vi "toggleShutter_v2.vi"(7 "Error In":errorcluster) -> (0 "error out":errorcluster)   [LabVIEW 2021]
doc: "Newport Motion Controler\nThis program Toggle Shutter (open / close)\n\nAndré Romero - 2020\nandretec@ifsc.usp.br"
uses:
  Global Shutter.vi
panel:
  out "VISA Refnum out":refnum<visa-resource-name>
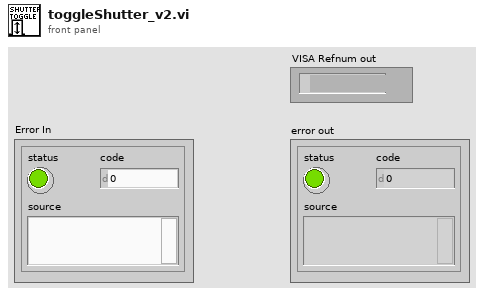
[diagram p1: front panel]
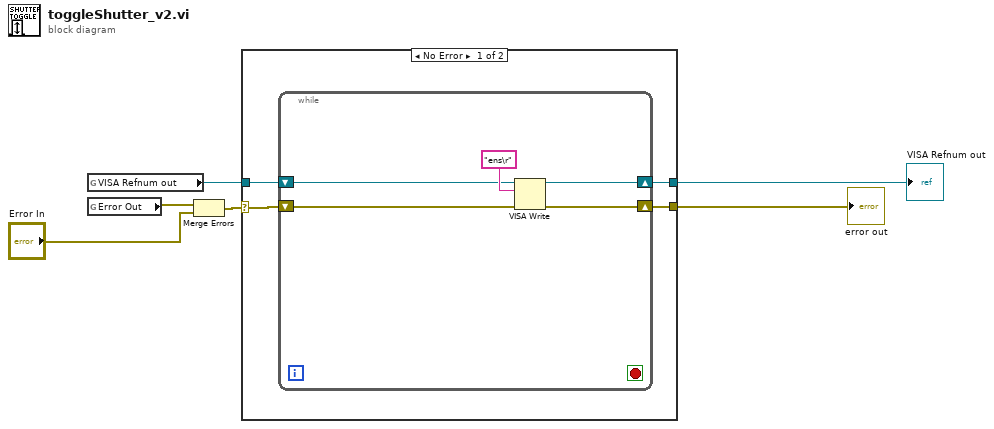
[diagram p0: block diagram]
diagram:
  n1 = global read "Global Shutter.vi" "VISA Refnum out"() -> (w4:refnum<visa-resource-name>)
  n2 = global read "Global Shutter.vi" "Error Out"() -> (w2:errorcluster)
  n3 = Merge Errors(w2, "Error In") -> (w3:errorcluster)
  n4 = case shown="No Error" w3 {
    selector: w3 -> [w7 w16]
    tunnel: [w10 w16] -> w6
    tunnel: [w9 w17] -> w5
    tunnel: w4 -> [w8 w17]
    frame No Error {
      n5 = while {
        shift-right: [w14] -> w9
        shift-left: w8 -> [w12]
        shift-right: [w15] -> w10
        shift-left: w7 -> [w11]
        stop <- _ stop-if-true
        n6 = VISA Write(VISA resource name=w12, write buffer="ens\r", error in (no error)=w11) -> (VISA resource name out=w14:refnum<visa-resource-name>, error out=w15:errorcluster)  [unwired: 1 out]
      }
    }
    frame Error {
    }
  }
  "error out" <- w6
  "VISA Refnum out" <- w5
